vi "Aula 02 - F para Celsius.vi"() -> ()   [LabVIEW 2024]
panel:
  in  "Numeric 3":dbl
  out "Numeric 2":i32
  in  "stop 2":bool
  in  "milliseconds to wait 2":u32
  in  "ºF 2":dbl(slide) scale=0.0..150.0 scale format="%#_2f"
  out "ºC 2":dbl(slide) scale=0.0..100.0 scale format="%#_2f"
  in  "Boolean":bool
  out "ºC":dbl(slide) scale=0.0..100.0 scale format="%#_2f"
  in  "ºF":dbl(slide) scale=0.0..150.0 scale format="%#_2f"
  in  "milliseconds to wait":u32
  in  "stop":bool
  out "Numeric":i32
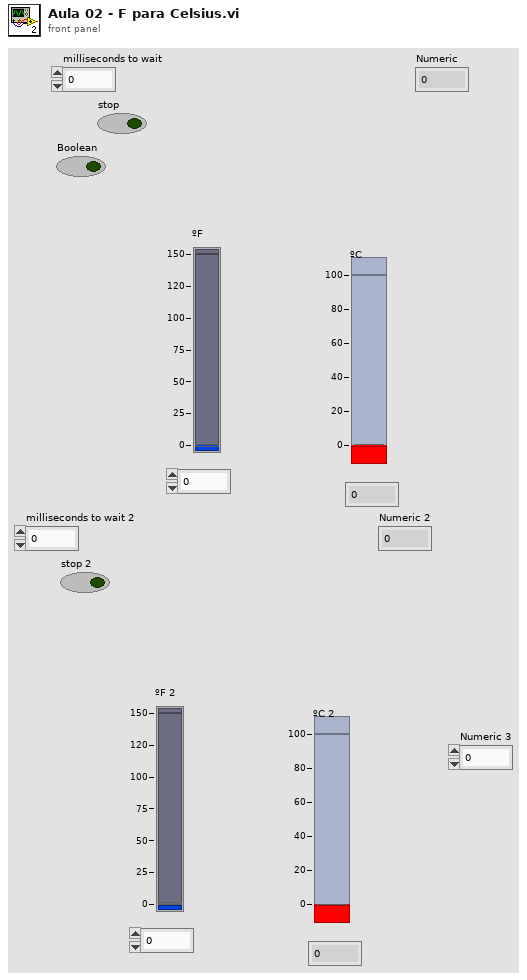
[diagram p1: front panel]
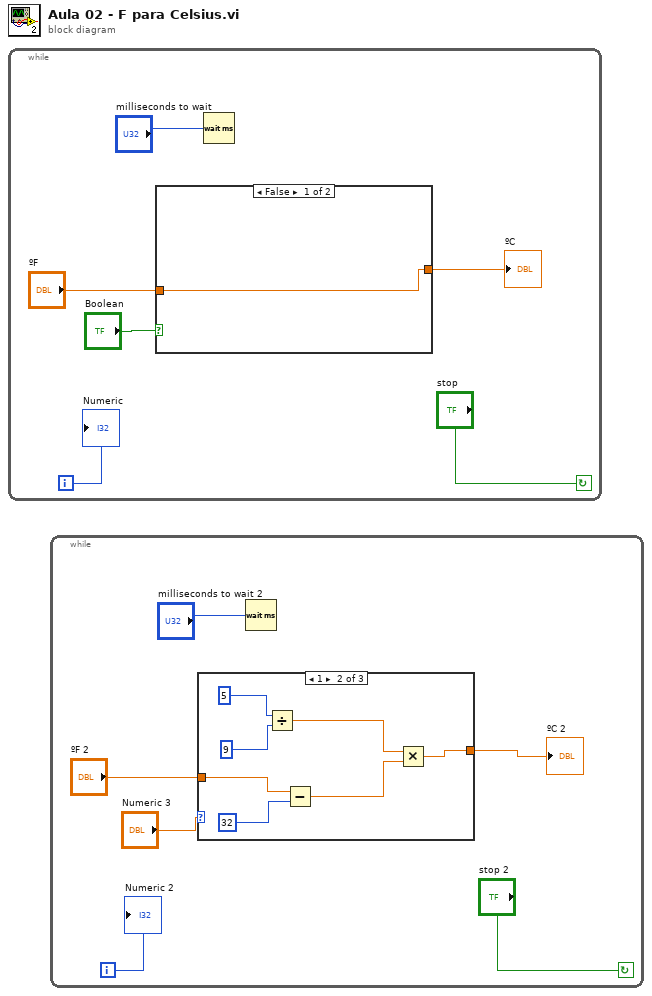
[diagram p0: block diagram]
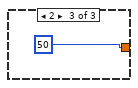
[diagram p3: hidden frame]
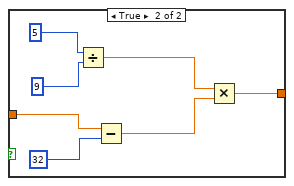
[diagram p4: hidden frame]
diagram:
  n1 = while {
    i -> [w6]
    stop <- "stop" continue-if-true
    n2 = case shown="False" "Boolean" {
      tunnel: "ºF" -> [w7 w10]
      tunnel: [w7 w8] -> w2
      frame False {
      }
      frame True {
        n3 = Divide(x=5, y=9) -> (x/y=w11:dbl)
        n4 = Subtract(x=w10, y=32) -> (x-y=w12:dbl)
        n5 = Multiply(x=w11, y=w12) -> (x*y=w8:dbl)
      }
    }
    "ºC" <- w2
    n6 = Wait (ms)(milliseconds to wait="milliseconds to wait") -> ()  [unwired: 1 out]
    "Numeric" <- w6
  }
  n7 = while {
    i -> [w20]
    stop <- "stop 2" continue-if-true
    n8 = case shown="1" "Numeric 3" {
      tunnel: "ºF 2" -> [w21 w24 _]
      tunnel: [w21 w22 50] -> w16
      frame 0, Default {
      }
      frame 1 {
        n9 = Divide(x=5, y=9) -> (x/y=w25:dbl)
        n10 = Subtract(x=w24, y=32) -> (x-y=w26:dbl)
        n11 = Multiply(x=w25, y=w26) -> (x*y=w22:dbl)
      }
      frame 2 {
      }
    }
    "ºC 2" <- w16
    n12 = Wait (ms)(milliseconds to wait="milliseconds to wait 2") -> ()  [unwired: 1 out]
    "Numeric 2" <- w20
  }
